vi "Get (PV Data).vi"(7 "PV name":string, 8 "error in":errorcluster, 9 "timeout":dbl[unit]=1.0, 11 "Client in":refnum<class "Client.lvclass">) -> (0 "error out":errorcluster, 1 "timed out?":bool, 2 "PV Data out":refnum<class "PV Data.lvclass">, 3 "Client out":refnum<class "Client.lvclass">)   [LabVIEW 2020, in "PV Access.lvlib" / "PVA Client.lvlib" / "Client.lvclass"]
uses:
  Client.lvclass
  PV Data/PV Data/PV Data.lvclass
  Client.lvclass/Client.ctl
  PV Access.lvlib
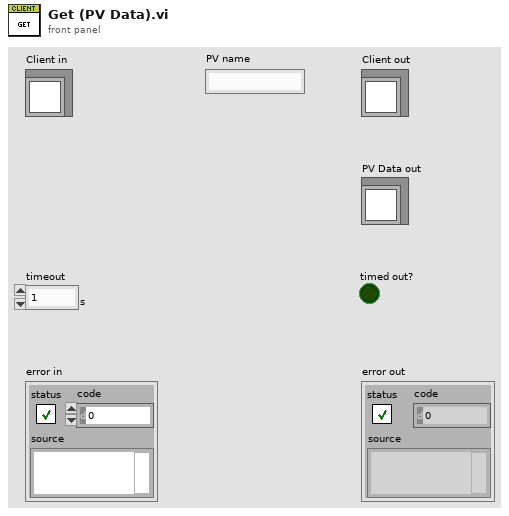
[diagram p1: front panel]
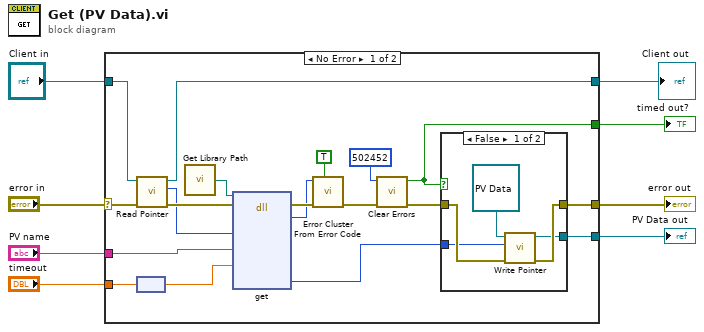
[diagram p0: block diagram]
diagram:
  n1 = case shown="No Error" "error in" {
    selector: "error in" -> [w27 w35]
    tunnel: [w11 w35] -> w5
    tunnel: [w22 w34] -> w4
    tunnel: "Client in" -> [w23 w34]
    tunnel: "PV name" -> [w24 _]
    tunnel: "timeout" -> [w19 _]
    tunnel: [w10 _] -> w1
    tunnel: [w9 _] -> w2
    frame No Error {
      n2 = call-dynamic "Read Pointer.vi"("error in (no error)"=w27, "Pointer Base in"=w23) -> ("error out"=w26:errorcluster, "Pointer"=w25:i64, "Pointer Base out"=w22:refnum<class "Client.lvclass">)  [unwired: 7 in]
      n3 = node(w19) -> (w20:dbl)
      n4 = call "Get Library Path.vi"() -> ("Path"=w21:path)  [unwired: 1 in]
      n5 = dll-call lib="?" fn="get"(path in=w21, error in=w26, "client"=w25, "pv_name"=w24, "timeout"=w20) -> (error out=w17:errorcluster, "ret_code"=w16:i32, "value"=w15:i64)  [unwired: 5 in, 1 out]
      n6 = call <vilib>:"Error Cluster From Error Code.vi"("show call chain? (False)"=TRUE, "error in (no error)"=w17, "error code (0)"=w16) -> ("error out"=w14:errorcluster)  [unwired: 6 in]
      n7 = call <vilib>:"Clear Errors.vi"("error in (no error)"=w14, "specific error code to clear (0: all)"=502452) -> ("error out"=w12:errorcluster, "specific error cleared?"=w9:bool)  [unwired: 4 in]
      n8 = case shown="False" w9 {
        tunnel: w15 -> [w29 _]
        tunnel: w12 -> [w32 w33]
        tunnel: [w31 w33] -> w11
        tunnel: [w30 _] -> w10
        frame False {
          n9 = call-dynamic "Write Pointer.vi"("error in (no error)"=w32, "Pointer"=w29, "Pointer Base in"=refnum<class "PV Data.lvclass"> refnum ("PV Access.lvlib:PV Data.lvlib:PV Data.lvclass")) -> ("error out"=w31:errorcluster, "Pointer Base out"=w30:refnum<class "PV Data.lvclass">)  [unwired: 7 in]
        }
        frame True {
        }
      }
    }
    frame Error {
    }
  }
  "error out" <- w5
  "Client out" <- w4
  "PV Data out" <- w1
  "timed out?" <- w2
